vi "Kicker.vi"(5 "IA State Input":T1={"our_robots"=[], "enemy_robots"=[], "balls"=[], "geometry"={"line_width"=0, "field_length"=0, "field_width"=0, "boundary_width"=0, "referee_width"=0, "goal_width"=0, "goal_depth"=0, "goal_wall_width"=0, "center_circle_radius"=0, "defense_radius"=0, "defense_stretch"=0, "free_kick_from_defense_dist"=0, "penalty_spot_from_field_line_dist"=0, "penalty_line_from_spot_dist"=0}, "IA Judge"={"stage"="", "command"="", "our_goalie_id"=0.0, "enemy_goalie_id"=0.0, "command enum"=enum."Halt", "Time"=enum."Azul"}, "Received Timestamp"=timestamp(0 s since 1904-01-01), "Events"={"Touch"=FALSE, "Ball out"=FALSE, "id touch"=0.0, "Ball out of \nVision"=FALSE, "Ball inside \nGoalie area"=FALSE, "Robot not responding"=FALSE, "Robots responding status"=[1.0, 1.0, 1.0, 1.0, 1.0, 1.0], "Enemy Ball \nPossession"=FALSE, "Pass State"=FALSE, "id end of pass"=0.0, "Kick"=FALSE, "Id ini Possession"=0.0, "Ball Possesion"=FALSE, "Id Possesion"=0.0}}, 6 "gravar":bool=TRUE, 7 "Dribble":bool, 8 "Ball velocity":dbl[](array[numeric]), 9 "Vel_kick":dbl=5.0 format="%#_13g", 10 "Kick?":bool, 11 "Robot in":T2={"id"=5, "function"=enum."Attacker", "x"=-983.1382446289062, "y"=-3000.010498046875, "orientation"=-1.5516623258590698, "v_tangent"=0.0, "v_normal"=0.0, "v_ang"=0.0, "kick_x"=0.0, "kick_z"=0.0, "dribble"=FALSE, "Timestamp"=timestamp(2082759045.994995 s since 1904-01-01), "dest_x"=0.0, "dest_y"=0.0, "dest_orientation"=0.0, "estimatives"={"est_v_tangent"=0.0, "est_v_normal"=0.0, "est_vx"=0.0, "est_vy"=0.0, "Pos Robot Est"=[]}, "dest_x_kick"=0.0, "dest_y_kick"=0.0, "Gap Coord"=[], "States"=enum."GoToTangent"}) -> (2 "output cluster":T2={"id"=0, "function"=enum."Attacker", "x"=0.0, "y"=0.0, "orientation"=0.0, "v_tangent"=0.0, "v_normal"=0.0, "v_ang"=0.0, "kick_x"=0.0, "kick_z"=0.0, "dribble"=FALSE, "Timestamp"=timestamp(0 s since 1904-01-01), "dest_x"=0.0, "dest_y"=0.0, "dest_orientation"=0.0, "estimatives"={"est_v_tangent"=0.0, "est_v_normal"=0.0, "est_vx"=0.0, "est_vy"=0.0, "Pos Robot Est"=[]}, "dest_x_kick"=0.0, "dest_y_kick"=0.0, "Gap Coord"=[], "States"=enum."GoToTangent"})   [LabVIEW 2017]
uses:
  Core/AI Robot.ctl
  Functions Enum.ctl
  AttackerStates.ctl
  Core/AI Input.ctl
  Core/AI Ball.ctl
  Core/Field Size.ctl
  Core/AI Judge.ctl
  Command Enum.ctl
  Util/Events/Events.ctl
panel:
  in  "file path (use dialog) 2":path=path "C:/temp/size.csv"
  in  "file path (use dialog)":path=path "C:/temp/chutes.csv"
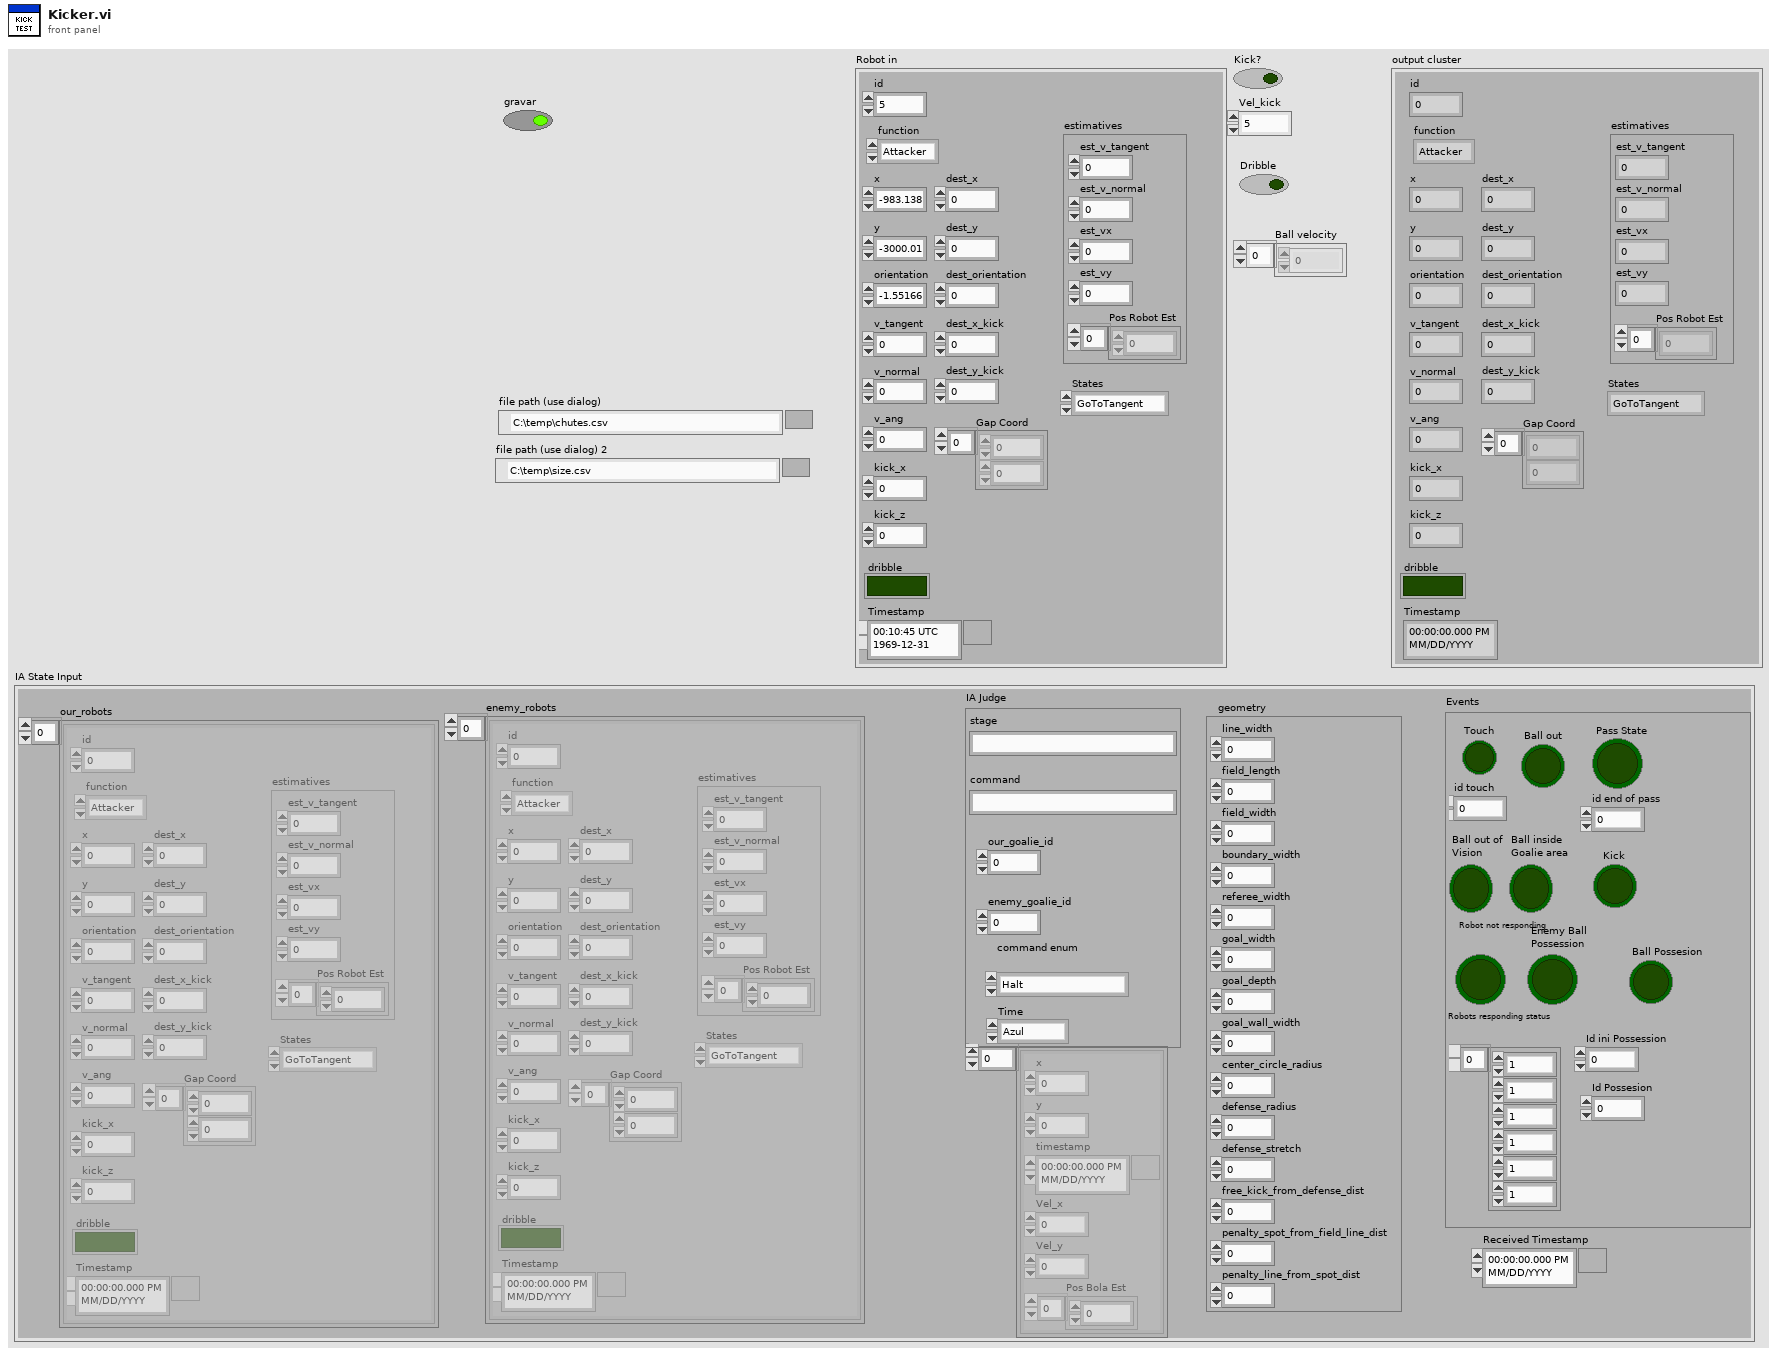
[diagram p1: front panel]
types:
  T1 = typedef "AI Input.ctl" = cluster{"our_robots":T2[], "enemy_robots":T2[], "balls":T5[], "geometry":T6, "IA Judge":T7, "Received Timestamp":timestamp, "Events":T9}
  T2 = typedef "AI Robot.ctl" = cluster{"id":u32, "function":T3, "x":dbl, "y":dbl, "orientation":dbl, "v_tangent":dbl, "v_normal":dbl, "v_ang":dbl, "kick_x":dbl, "kick_z":dbl, "dribble":bool, "Timestamp":timestamp, "dest_x":dbl, "dest_y":dbl, "dest_orientation":dbl, "estimatives":cluster{"est_v_tangent":dbl, "est_v_normal":dbl, "est_vx":dbl, "est_vy":dbl, "Pos Robot Est":dbl[]}, "dest_x_kick":dbl, "dest_y_kick":dbl, "Gap Coord":dbl[], "States":T4}
  T3 = typedef "Functions Enum.ctl" = enum16{"Attacker", "Goalie", "Defender", "Striker", "Goto 0", "Dummy", "Kicker", "ZigZag"}
  T4 = typedef "AttackerStates.ctl" = enum16{"Pass", "GoToTangent", "BallGetting", "GoToKick", ""}
  T5 = typedef "AI Ball.ctl" = cluster{"x":dbl, "y":dbl, "timestamp":timestamp, "Vel_x":dbl, "Vel_y":dbl, "Pos Bola Est":dbl[]}
  T6 = typedef "Field Size.ctl" = cluster{"line_width":u32, "field_length":u32, "field_width":u32, "boundary_width":u32, "referee_width":u32, "goal_width":u32, "goal_depth":u32, "goal_wall_width":u32, "center_circle_radius":u32, "defense_radius":u32, "defense_stretch":u32, "free_kick_from_defense_dist":u32, "penalty_spot_from_field_line_dist":u32, "penalty_line_from_spot_dist":u32}
  T7 = typedef "AI Judge.ctl" = cluster{"stage":string, "command":string, "our_goalie_id":dbl, "enemy_goalie_id":dbl, "command enum":T8, "Time":enum16{"Azul", "Amarelo"}}
  T8 = typedef "Command Enum.ctl" = enum16{"Halt", "Stop", "Force Start", "PKA Normal Start", "Prepare Kickoff Ally", "PKE Normal Start", "Prepare Kickoff Enemy", "Prepare Penalty Ally", "PPA Normal Start", "Prepare Penalty Enemy", "PPE Normal Start", "Direct Free Enemy", "Direct Free Ally", "Indirect Free Enemy", "Indirect Free Ally", "Timeout Enemy", "Timeout Ally", "Goal Enemy", "Goal Ally", "Ball Placement Enemy", "Ball Placement Ally", "Normal Half Time", "Extra Time Break", "Extra Half Time", "None", "Post Game"}
  T9 = typedef "Events.ctl" = cluster{"Touch":bool, "Ball out":bool, "id touch":dbl, "Ball out of \nVision":bool, "Ball inside \nGoalie area":bool, "Robot not responding":bool, "Robots responding status":dbl[], "Enemy Ball \nPossession":bool, "Pass State":bool, "id end of pass":dbl, "Kick":bool, "Id ini Possession":dbl, "Ball Possesion":bool, "Id Possesion":dbl}
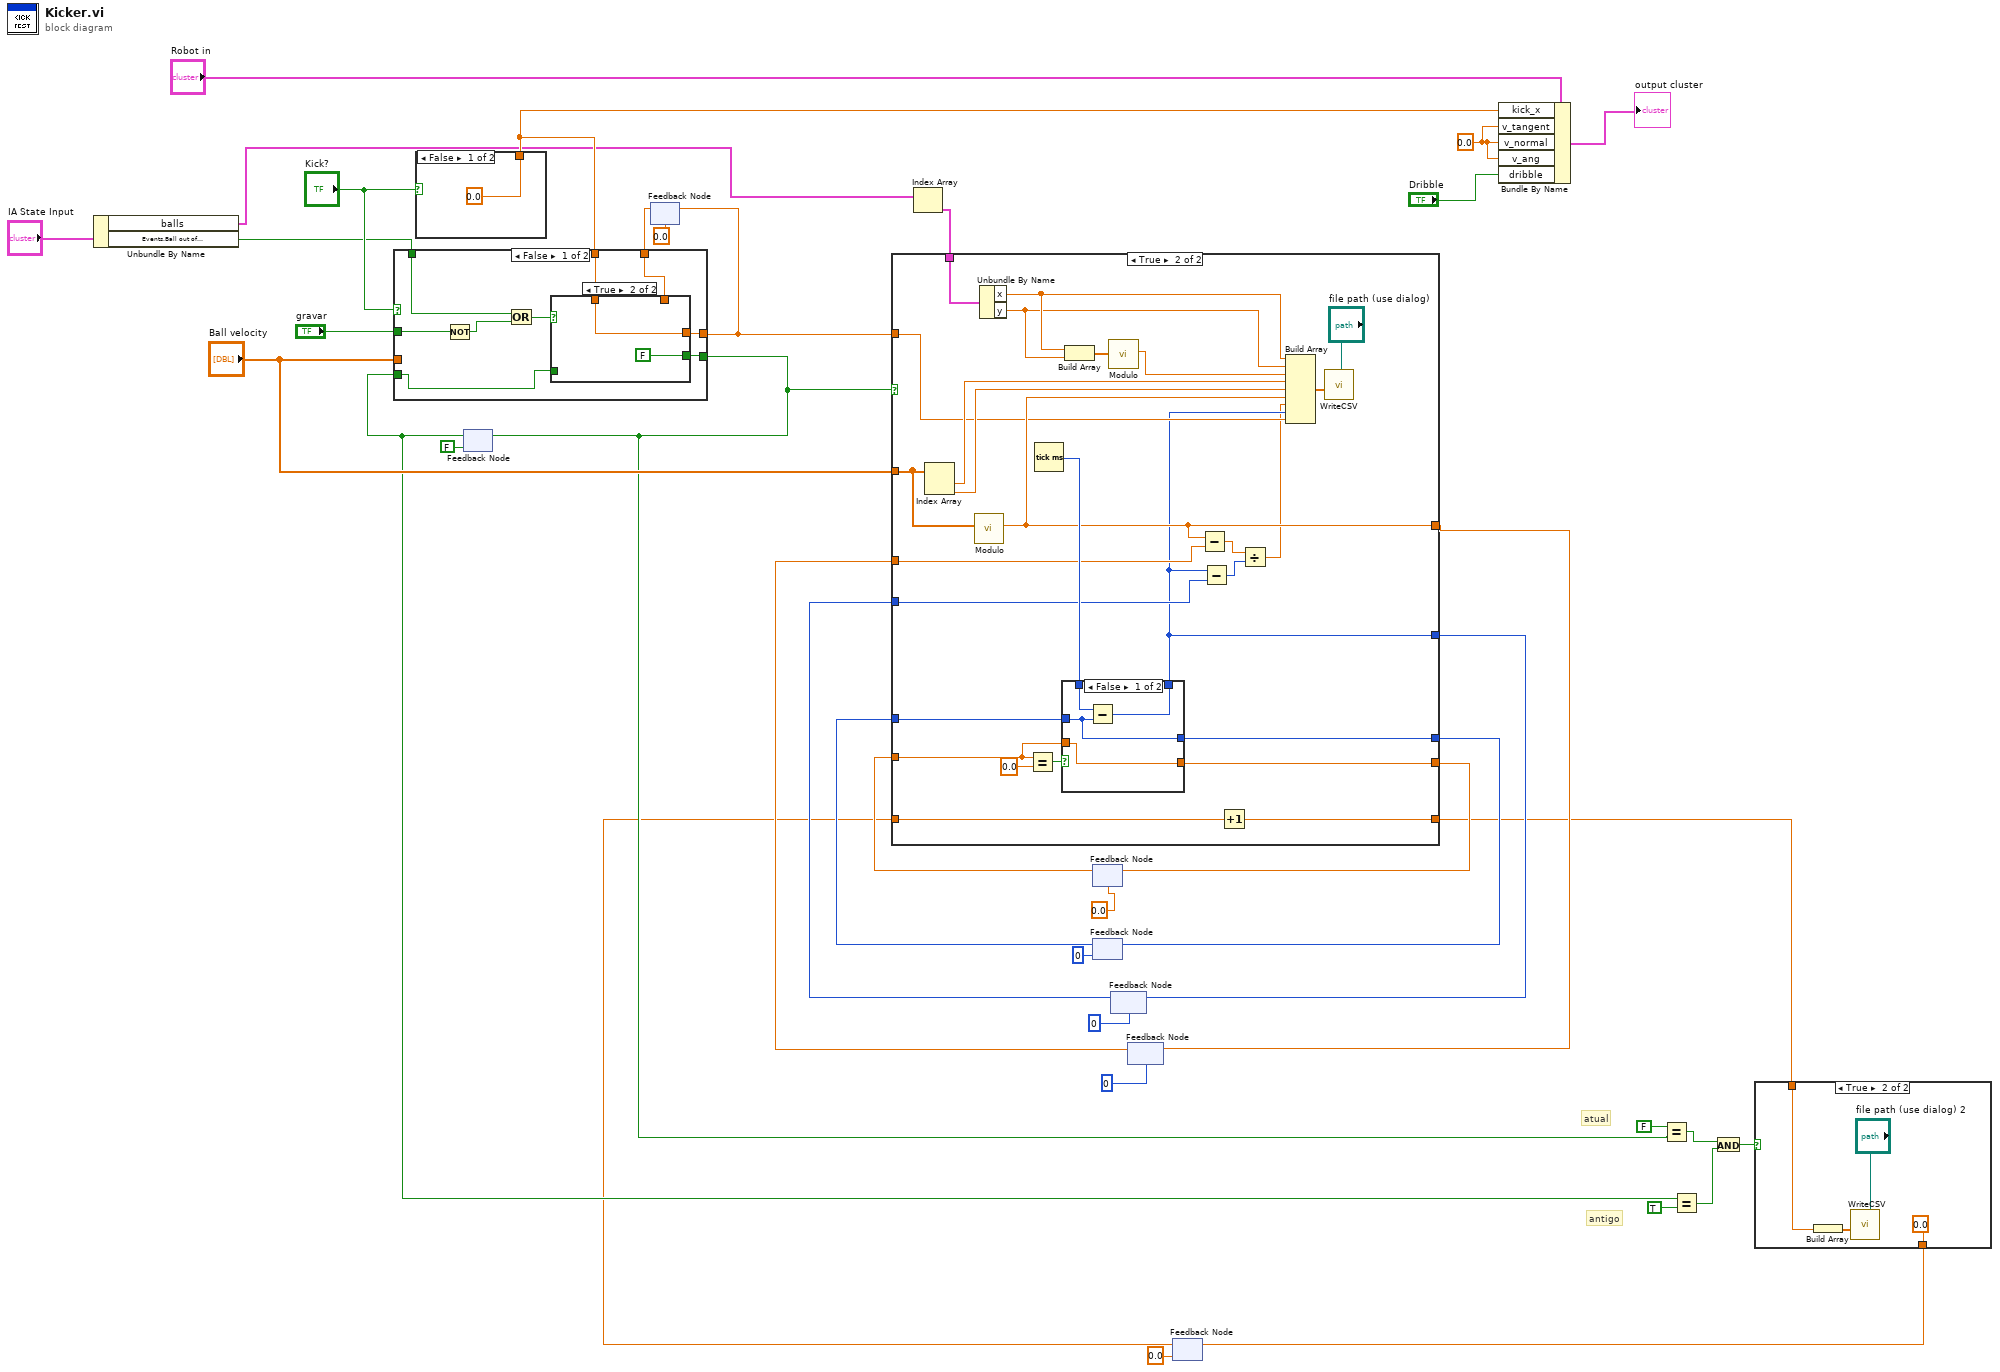
[diagram p0: block diagram]
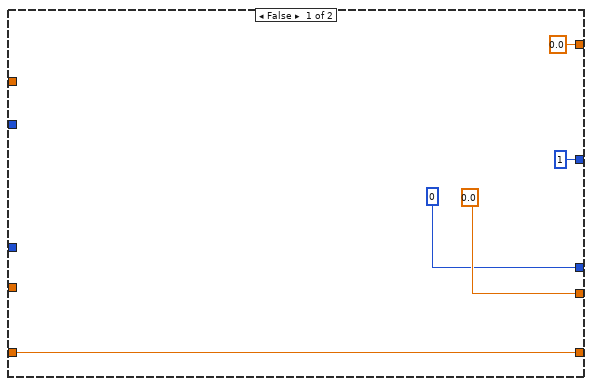
[diagram p3: hidden frame]
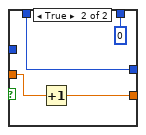
[diagram p4: hidden frame]
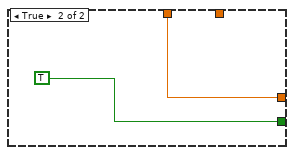
[diagram p6: hidden frame]
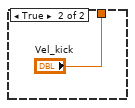
[diagram p7: hidden frame]
diagram:
  w37 = 0.0 ("v_normal")
  # "antigo"
  # "atual"
  n1 = Unbundle By Name("IA State Input") -> ("balls"=w13:T5[], "Events.Ball out of \nVision"=w33:bool)
  n2 = case shown="False" "Kick?" {
    tunnel: [0.0 "Vel_kick"] -> w30
    frame False {
    }
    frame True {
    }
  }
  n3 = feedback #1(FALSE) -> (w10:bool)
  n4 = feedback #2(0.0 ("Vel_kick")) -> (w29:dbl)
  n5 = case shown="False" "Kick?" {
    tunnel: [w48 TRUE] -> w11
    tunnel: w10 -> [w47 _]
    tunnel: "Ball velocity" -> [_ _]
    tunnel: w33 -> [w49 _]
    tunnel: w30 -> [w45 w55]
    tunnel: [w46 w55] -> w27
    tunnel: w29 -> [w44 _]
    tunnel: "gravar" -> [w42 _]
    frame False {
      n6 = Not(x=w42) -> (.not. x?=w43:bool)
      n7 = Or(x=w49, y=w43) -> (x .or. y?=w50:bool)
      n8 = case shown="True" w50 {
        tunnel: [w52 FALSE] -> w48
        tunnel: w47 -> [w52 _]
        tunnel: [w51 w53] -> w46
        tunnel: w45 -> [_ w53]
        tunnel: w44 -> [w51 _]
        frame False {
        }
        frame True {
        }
      }
    }
    frame True {
    }
  }
  n9 = feedback-in #1(w11) -> ()
  n10 = feedback-in #2(w27) -> ()
  n11 = Index Array(array=w13) -> (element=w14:T5)  [unwired: 1 in]
  n12 = feedback #3(0.0) -> (w25:dbl)
  n13 = feedback #4(u32 0 ("millisecond timer value")) -> (w22:u32)
  n14 = feedback #5(u32 0 ("millisecond timer value")) -> (w19:u32)
  n15 = feedback #6(u32 0 ("millisecond timer value")) -> (w17:dbl)
  n16 = feedback #7(0.0) -> (w2:dbl)
  n17 = case shown="True" w11 {
    tunnel: "Ball velocity" -> [_ w84]
    tunnel: w27 -> [_ w71]
    tunnel: [0.0 w82] -> w26
    tunnel: w25 -> [_ w79]
    tunnel: [u32 0 ("millisecond timer value") w77] -> w23
    tunnel: w22 -> [_ w78]
    tunnel: [u32 1 w70] -> w20
    tunnel: w19 -> [_ w74]
    tunnel: [0.0 ("Modulo") w76] -> w18
    tunnel: w17 -> [_ w75]
    tunnel: w14 -> [_ w68]
    tunnel: [w57 w63] -> w3
    tunnel: w2 -> [w57 w62]
    frame False {
    }
    frame True {
      n18 = Index Array(array=w84) -> (element #1=w88:dbl, element #2=w85:dbl)  [unwired: 2 in]
      n19 = call "Modulo.vi"("2D vector"=w84) -> ("Modulo"=w76:dbl)  [unwired: 10 in]
      n20 = Unbundle By Name(w68) -> ("x"=w67:dbl, "y"=w66:dbl)
      n21 = Equal?(x=w79, y=0.0) -> (x = y?=w81:bool)
      n22 = Tick Count (ms)() -> (millisecond timer value=w83:u32)
      n23 = case shown="False" w81 {
        tunnel: w83 -> [w92 w94]
        tunnel: [w91 w96] -> w82
        tunnel: w79 -> [w91 w95]
        tunnel: [w90 w94] -> w77
        tunnel: w78 -> [w90 _]
        tunnel: [w89 u32 0] -> w70
        frame False {
          n24 = Subtract(x=w92, y=w90) -> (x-y=w89:u32)
        }
        frame True {
          n25 = Increment(x=w95) -> (x+1=w96:dbl)
        }
      }
      n26 = Build Array(w67, w66) -> (w65:dbl[])
      n27 = call "Modulo.vi"("2D vector"=w65) -> ("Modulo"=w64:dbl)  [unwired: 10 in]
      n28 = Subtract(x=w76, y=w75) -> (x-y=w73:dbl)
      n29 = Subtract(x=w70, y=w74) -> (x-y=w72:u32)
      n30 = Increment(x=w62) -> (x+1=w63:dbl)
      n31 = Divide(x=w73, y=w72) -> (x/y=w69:dbl)
      n32 = Build Array(w67, w66, w64, w88, w85, w76, w69, w70, w71) -> (w87:dbl[])
      n33 = call "WriteCSV.vi"("array"=w87, "file path (use dialog)"="file path (use dialog)") -> ()  [unwired: 10 in]
    }
  }
  n34 = feedback-in #3(w26) -> ()
  n35 = feedback-in #4(w23) -> ()
  n36 = feedback-in #5(w20) -> ()
  n37 = feedback-in #6(w18) -> ()
  n38 = Bundle By Name(cluster="Robot in", "kick_x"=w30, "v_tangent"=w37, "v_normal"=w37, "v_ang"=w37, "dribble"="Dribble") -> (→"output cluster":T2)
  n39 = Equal?(x=FALSE, y=w11) -> (x = y?=w6:bool)
  n40 = Equal?(x=w10, y=TRUE) -> (x = y?=w5:bool)
  n41 = And(x=w6, y=w5) -> (x .and. y?=w7:bool)
  n42 = case shown="True" w7 {
    tunnel: [w97 0.0] -> w4
    tunnel: w3 -> [w97 w99]
    frame False {
    }
    frame True {
      n43 = Build Array(w99) -> (w100:dbl[])
      n44 = call "WriteCSV.vi"("array"=w100, "file path (use dialog)"="file path (use dialog) 2") -> ()  [unwired: 10 in]
    }
  }
  n45 = feedback-in #7(w4) -> ()
